vi "File.Remove Empty SubDirs.vi"(11 "Dir":path) -> (3 "Deleted":path[](array[path]))   [LabVIEW 2018]
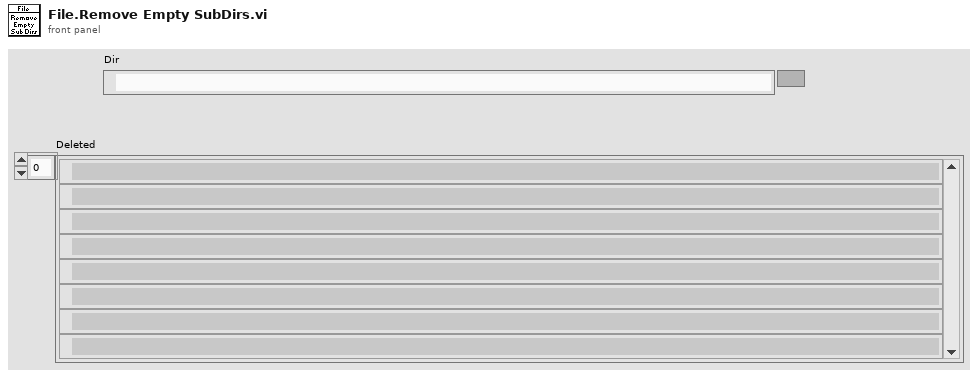
[diagram p1: front panel]
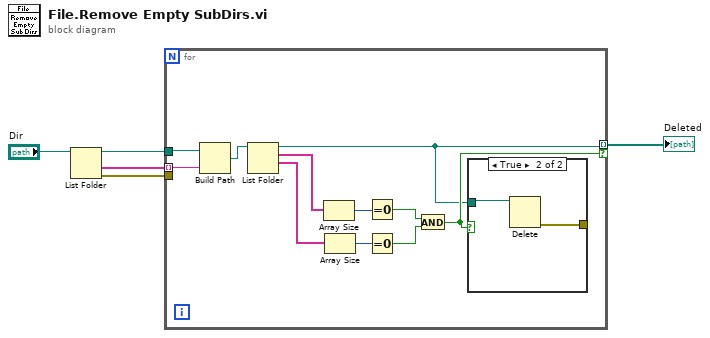
[diagram p0: block diagram]
diagram:
  n1 = List Folder(path="Dir") -> (path out=w4:path, folder names=w3:string[], error out=w1:errorcluster)  [unwired: 3 in, 1 out]
  n2 = for {
    tunnel: w4 -> [w15]
    tunnel: w3 -> [w16] mode=indexing
    tunnel: [w6] -> w2 mode=indexing if=w7
    tunnel: w1 -> [_]
    n3 = Build Path(base path=w15, name or relative path=w16) -> (appended path=w14:path)
    n4 = List Folder(path=w14) -> (path out=w6:path, filenames=w13:string[], folder names=w12:string[])  [unwired: 3 in, 1 out]
    n5 = Array Size(array=w13) -> (size(s)=w11:i32)
    n6 = Array Size(array=w12) -> (size(s)=w10:i32)
    n7 = Equal To 0?(x=w11) -> (x = 0?=w9:bool)
    n8 = Equal To 0?(x=w10) -> (x = 0?=w8:bool)
    n9 = And(x=w9, y=w8) -> (x .and. y?=w7:bool)
    n10 = case shown="True" w7 {
      tunnel: w6 -> [_ w18]
      tunnel: [_ w17] -> _
      frame False {
      }
      frame True {
        n11 = Delete(path (use dialog)=w18) -> (error out=w17:errorcluster)  [unwired: 4 in, 2 out]
      }
    }
  }
  "Deleted" <- w2
